vi "RoboRealm.vi"(3 "error in (no error)":errorcluster, 4 "connection ID IN":refnum<k5>, 5 "Max Variable Length":i32 step=7, 6 "Variable Name":string) -> (0 "error out":errorcluster, 1 "Variable Value":string, 2 "connection ID out":refnum<k5>)   [LabVIEW 2019]
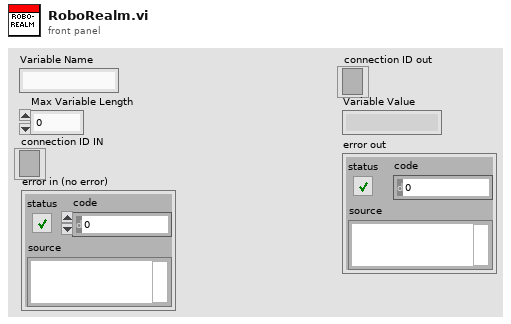
[diagram p1: front panel]
types:
  T1 = enum16{"Standard", "Buffered", "CRLF", "Immediate"}
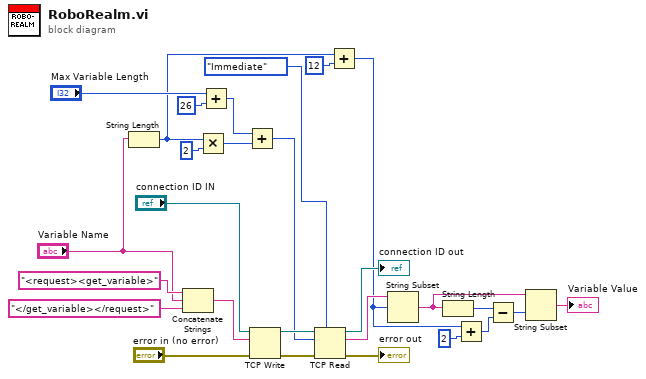
[diagram p0: block diagram]
diagram:
  n1 = String Length(string="Variable Name") -> (length=w13:i32)
  n2 = Concatenate Strings("<request><get_variable>" ("string"), "Variable Name", "</get_variable></request>" ("string")) -> (w19:string)
  n3 = Multiply(x=w13, y=2) -> (x*y=w21:i32)
  n4 = Add(x="Max Variable Length", y=26) -> (x+y=w24:i32)
  n5 = Add(x=w24, y=w21) -> (x+y=w17:i32)
  n6 = TCP Write(connection ID="connection ID IN", data in=w19, error in (no error)="error in (no error)") -> (connection ID out=w18:refnum<k5>, error out=w2:errorcluster)  [unwired: 1 in, 1 out]
  n7 = TCP Read(connection ID=w18, bytes to read=w17, error in (no error)=w2, 7:T1."Immediate" ("mode (standard)")) -> (connection ID out=→"connection ID out":refnum<k5>, data out=w11:string, error out=→"error out":errorcluster)  [unwired: 1 in]
  n8 = Add(x=w13, y=12) -> (x+y=w10:i32)
  n9 = String Subset(string=w11, offset (0)=w10) -> (substring=w6:string)  [unwired: 1 in]
  n10 = String Length(string=w6) -> (length=w8:i32)
  n11 = Add(x=w10, y=2) -> (x+y=w7:i32)
  n12 = Subtract(x=w8, y=w7) -> (x-y=w1:i32)
  n13 = String Subset(string=w6, length (rest)=w1) -> (substring=→"Variable Value":string)  [unwired: 1 in]
